vi "Read PID.vi"(8 "error in (no error)":errorcluster, 11 "Humidifier in":refnum<class "Humidifier.lvclass">) -> (0 "error out":errorcluster, 2 "PID":cluster{"P":sgl, "I":sgl, "D":sgl}, 3 "Humidifier out":refnum<class "Humidifier.lvclass">)   [LabVIEW 2014, in "Humidifier Lib.lvlib" / "Humidifier.lvclass"]
uses:
  Humidifier.lvclass
  Humidifier.lvclass/Humidifier.ctl
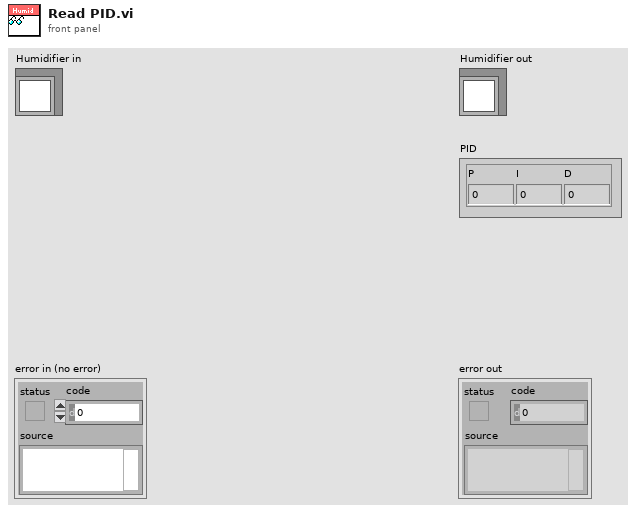
[diagram p1: front panel]
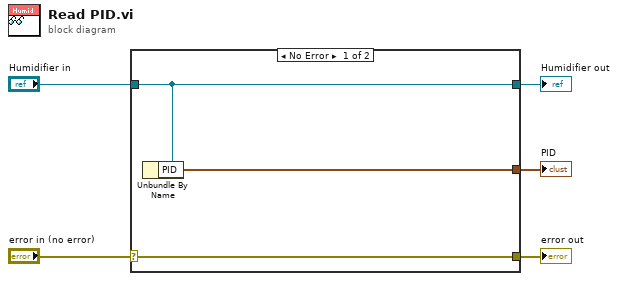
[diagram p0: block diagram]
diagram:
  n1 = case shown="No Error" "error in (no error)" {
    selector: "error in (no error)" -> [w8 w9]
    tunnel: [w8 w9] -> w4
    tunnel: [w7 w10] -> w2
    tunnel: "Humidifier in" -> [w7 w10]
    tunnel: [w6 _] -> w1
    frame No Error {
      n2 = Unbundle By Name(w7) -> ("PID"=w6:cluster{"P":sgl, "I":sgl, "D":sgl})
    }
    frame Error {
    }
  }
  "error out" <- w4
  "Humidifier out" <- w2
  "PID" <- w1
